vi "Measurement Logic.vi"(8 "error in":errorcluster, 9 "measurement configuration":T2, 10 "measure call context in":refnum<class "Measure Call Context.lvclass">, 11 "Stop OOB Server UE":refnum<user-event>) -> (0 "error out":errorcluster, 1 "measurement results":T1 {"Scanned Addresses" format="%.0x"}, 2 "measure call context out":refnum<class "Measure Call Context.lvclass">)   [LabVIEW 2025, in "I2C Bus Monitor.lvclass"]
doc: "Contains the core logic for executing the measurement."
uses:
  I2C Bus Monitor.lvclass
  <vilib>/Plug-In SDKs/Measurements/Measure Call Context/Measure Call Context.lvclass
  Measurement Configuration.ctl
  Measurement Results.ctl
  Typedefs/Logic Data.ctl
  Typedefs/State.ctl
  <instrlib>/FlexRIO/CSI-2/v2/FPGA/Types/Timestamp ID.ctl
  SubVIs/I2C Message Buffer - Create.vi
  SubVIs/I2C Message Buffer - Enqueue.vi
  SubVIs/I2C Message Buffer - Check.vi
  SubVIs/Error Global.vi
  SubVIs/I2C Message Buffer - Destroy.vi
  OOB Data Transfer/OOB Data Transfer.lvlib
  <instrlib>/_niInstr/Basic Elements/v1/FPGA/niInstr Basic Elements v1 FPGA.lvlib
  <instrlib>/FlexRIO/CSI-2/v2/FPGA/NI CSI-2 API FPGA v2.lvlib
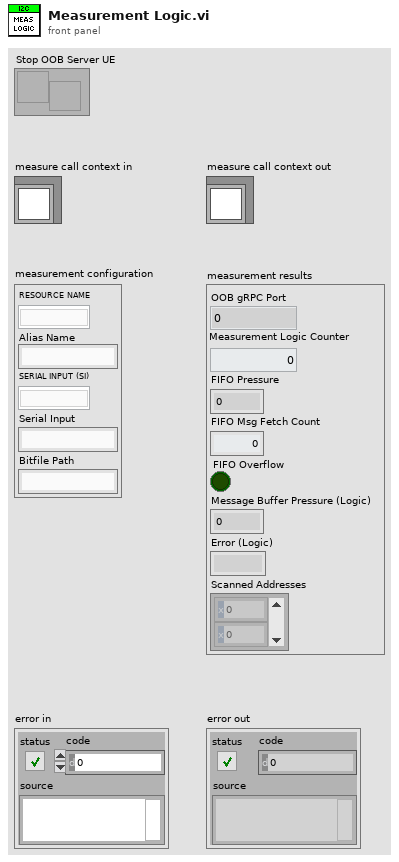
[diagram p1: front panel]
types:
  T1 = typedef "I2C Bus Monitor.lvclass/Measurement Results.ctl" = cluster{"OOB gRPC Port":i32, "Measurement Logic Counter":i32, "FIFO Pressure":u32, "FIFO Msg Fetch Count":i32, "FIFO Overflow":bool, "Message Buffer Pressure (Logic)":i32, "Error (Logic)":string, "Scanned Addresses":i32[]}
  T2 = typedef "I2C Bus Monitor.lvclass/Measurement Configuration.ctl" = cluster{"RESOURCE NAME":u32, "Alias Name":string, "SERIAL INPUT (SI)":u32, "Serial Input":string, "Bitfile Path":string}
  T3 = typedef "I2C Bus Monitor.lvclass/Logic Data.ctl" = cluster{"State":T4, "FPGA Ref":refnum<k20>, "Timestamp ID":T5, "Results":T1}
  T4 = typedef "I2C Bus Monitor.lvclass/State.ctl" = enum16{"Init", "Exec", "Results", "Error", "Close"}
  T5 = typedef "NI CSI-2 API FPGA v2.lvlib/Timestamp ID.ctl" = enum8{"SI0 LLP", "SI1 LLP", "SI2 LLP", "SI3 LLP", "SI4 LLP", "SI5 LLP", "SI6 LLP", "SI7 LLP", "SO0 LLP", "SO1 LLP", "SO2 LLP", "SO3 LLP", "SO4 LLP", "SO5 LLP", "SO6 LLP", "SO7 LLP", "Ser0 GPIO Bank", "Ser1 GPIO Bank", "Ser2 GPIO Bank", "Ser3 GPIO Bank", "Ser4 GPIO Bank", "Ser5 GPIO Bank", "Ser6 GPIO Bank", "Ser7 GPIO Bank", "Des0 GPIO Bank", "Des1 GPIO Bank", "Des2 GPIO Bank", "Des3 GPIO Bank", "Des4 GPIO Bank", "Des5 GPIO Bank", "Des6 GPIO Bank", "Des7 GPIO Bank", "User0", "User1", "User2", "User3", "User4", "User5", "User6", "User7", "User8", "User9", "User10", "User11", "User12", "User13", "User14", "User15", "User16", "User17", "User18", "User19", "User20", "User21", "User22", "User23", "User24", "User25", "User26", "User27", "User28", "User29", "User30", "User31"}
  T6 = typedef "OOB Data Transfer.lvlib/OOB to Logic Data.ctl" = cluster{"PauseResume":bool, "Export":string, "Scan Bus":bool, "I2C Script":cluster{"Send":bool, "Path":string}, "I2C CMD":cluster{"Send":bool, "SLAVE ADDR.":u8, "REG. ADDR.":u16, "DATA":u8, "R/W":bool}}
  T7 = cluster{"Send":bool, "SLAVE ADDR.":u8, "REG. ADDR.":u16, "DATA":u8, "R/W":bool}
  T8 = cluster{"Serial Input":string, "SLAVE ADDR.":u8, "REG. ADDR.":u16, "DATA":u8, "R/W":bool}
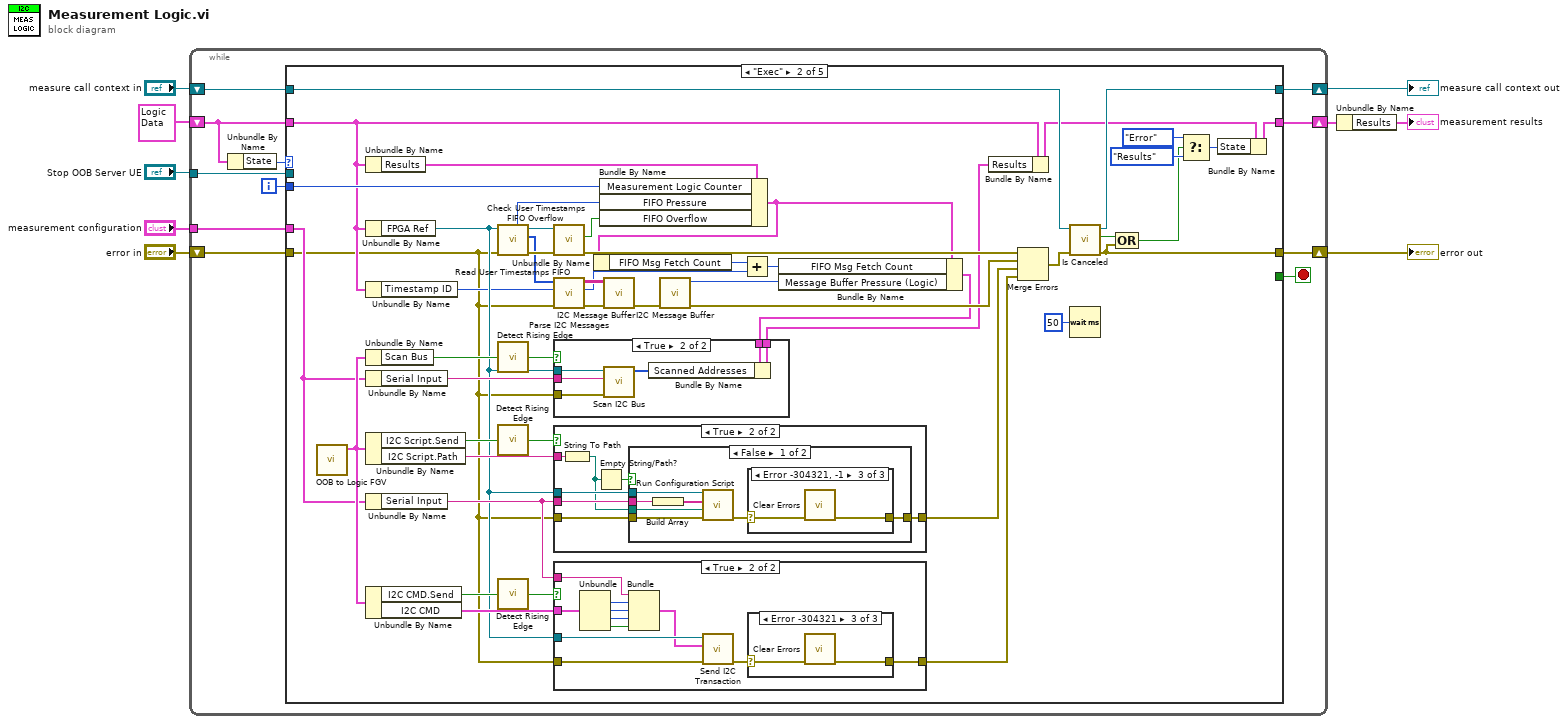
[diagram p0: block diagram]
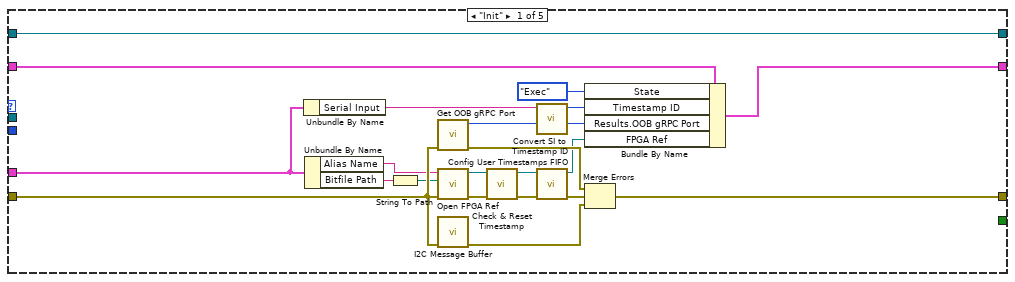
[diagram p2: hidden frame]
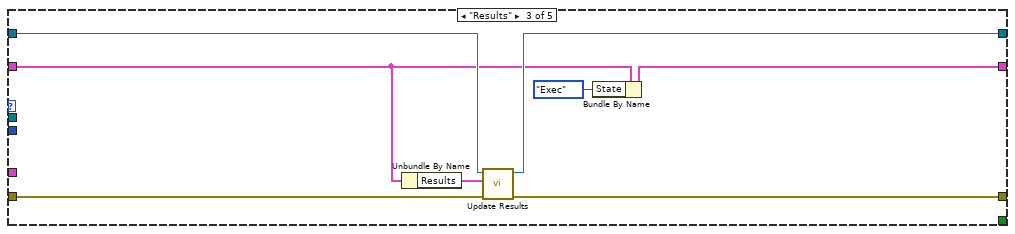
[diagram p11: hidden frame]
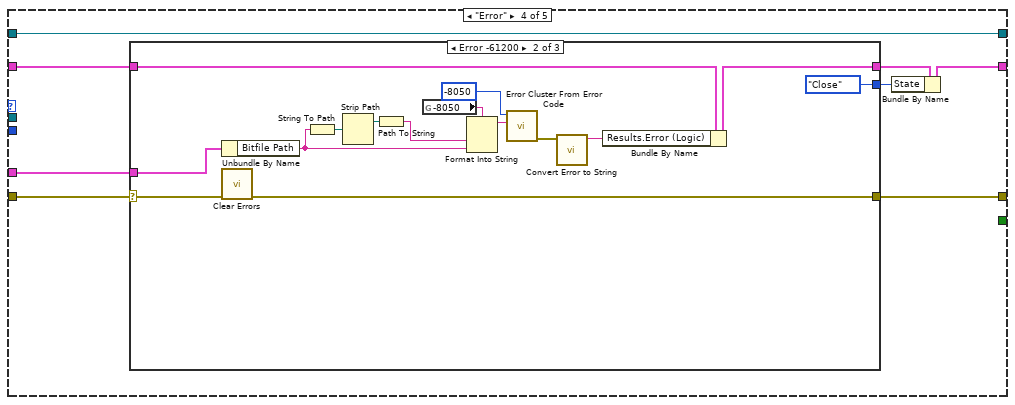
[diagram p12: hidden frame]
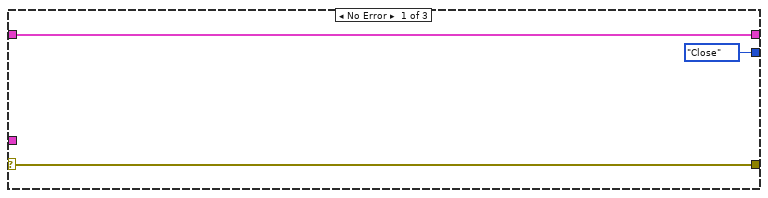
[diagram p13: hidden frame]
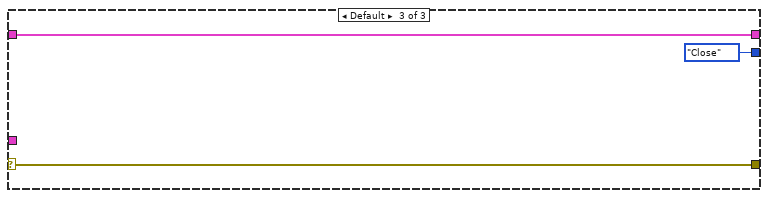
[diagram p14: hidden frame]
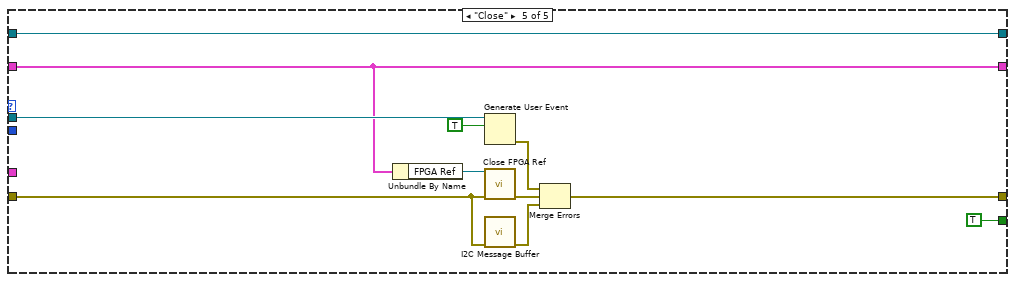
[diagram p15: hidden frame]
diagram:
  n1 = while {
    shift-right: [w15] -> w2
    shift-left: T3 {"State"=enum."Init", "FPGA Ref"=refnum, "Timestamp ID"=enum."SI0 LLP", "Results"={"OOB gRPC Port"=0, "Measurement Logic Counter"=0, "FIFO Pressure"=0, "FIFO Msg Fetch Count"=0, "FIFO Overflow"=FALSE, "Message Buffer Pressure (Logic)"=0, "Error (Logic)"="", "Scanned Addresses"=[]}} -> [w14]
    shift-right: [w10] -> w3
    shift-left: "error in" -> [w20]
    tunnel: "Stop OOB Server UE" -> [w18]
    tunnel: "measurement configuration" -> [w16]
    shift-right: [w11] -> w5
    shift-left: "measure call context in" -> [w17]
    i -> [w12]
    stop <- w19 stop-if-true
    n2 = Unbundle By Name(w14) -> ("State"=w13:T4)
    n3 = case shown="\"Exec\"" w13 {
      tunnel: w20 -> [w40 w44 w139 w148 w175]
      tunnel: [_ _ _ _ TRUE] -> w19
      tunnel: w18 -> [_ _ _ _ w179]
      tunnel: w17 -> [w22 w77 w137 w142 w180]
      tunnel: w16 -> [w25 w68 _ w143 _]
      tunnel: w14 -> [w39 w46 w135 w149 w171]
      tunnel: [w38 w79 w141 w145 w171] -> w15
      tunnel: w12 -> [_ w66 _ _ _]
      tunnel: [w26 w70 w138 w147 w174] -> w10
      tunnel: [w22 w76 w136 w142 w180] -> w11
      frame "Init" {
        n4 = Unbundle By Name(w25) -> ("Serial Input"=w36:string)
        n5 = Unbundle By Name(w25) -> ("Alias Name"=w31:string, "Bitfile Path"=w32:string)
        n6 = String To Path(string=w32) -> (path=w33:path)
        n7 = call "Get OOB gRPC Port.vi"("error in (no error)"=w40) -> ("error out"=w41:errorcluster, "OOB gRPC Port"=w21:i32)  [unwired: 9 in]
        n8 = call "Open FPGA Ref.vi"("error in (no error)"=w40, "Bitfile Path"=w33, "Device address"=w31) -> ("error out"=w34:errorcluster, "FPGA Ref out"=w29:refnum<k20>)  [unwired: 7 in]
        n9 = call-poly "I2C Message Buffer.vi"("error in (no error)"=w40) -> ("error out"=w27:errorcluster)  [unwired: 10 in]
        n10 = call "Check & Reset Timestamp.vi"("error in (no error)"=w34, "FPGA Ref in"=w29) -> ("error out"=w35:errorcluster, "FPGA Ref out"=w30:refnum<k20>)  [unwired: 8 in]
        n11 = call "Convert SI to Timestamp ID.vi"("SI Channel"=w36) -> ("Timestamp ID"=w23:T5)  [unwired: 10 in]
        n12 = call "Config User Timestamps FIFO.vi"("error in (no error)"=w35, "FPGA Ref in"=w30) -> ("error out"=w28:errorcluster, "FPGA Ref out"=w24:refnum<k20>)  [unwired: 8 in]
        n13 = Bundle By Name(cluster=w39, "State"=State."Exec", "Timestamp ID"=w23, "Results.OOB gRPC Port"=w21, "FPGA Ref"=w24) -> (w38:T3)
        n14 = Merge Errors(w41, w28, w27) -> (w26:errorcluster)
      }
      frame "Exec" {
        n15 = call "OOB to Logic FGV.vi"() -> ("OOB to Logic Data out"=w83:T6)  [unwired: 10 in, 1 out]
        n16 = Unbundle By Name(w46) -> ("Results"=w47:T1)
        n17 = Unbundle By Name(w46) -> ("FPGA Ref"=w60:refnum<k20>)
        n18 = Unbundle By Name(w46) -> ("Timestamp ID"=w53:T5)
        n19 = Unbundle By Name(w83) -> ("Scan Bus"=w61:bool)
        n20 = Unbundle By Name(w68) -> ("Serial Input"=w62:string)
        n21 = Unbundle By Name(w83) -> ("I2C Script.Send"=w88:bool, "I2C Script.Path"=w87:string)
        n22 = Unbundle By Name(w68) -> ("Serial Input"=w75:string)
        n23 = Unbundle By Name(w83) -> ("I2C CMD.Send"=w85:bool, "I2C CMD"=w82:T7)
        n24 = call "Read User Timestamps FIFO.vi"("error in (no error)"=w44, "FPGA Ref in"=w60) -> ("error out"=w90:errorcluster, "Data"=w54:u64[], "FPGA Ref out"=w81:refnum<k20>, "Elements Remaining"=w65:u32)  [unwired: 6 in]
        n25 = call <instrlib>:"Detect Rising Edge.vi"("signal"=w61) -> ("edge detected"=w51:bool)  [unwired: 14 in]
        n26 = call <instrlib>:"Detect Rising Edge.vi"("signal"=w88) -> ("edge detected"=w86:bool)  [unwired: 14 in]
        n27 = call <instrlib>:"Detect Rising Edge.vi"("signal"=w85) -> ("edge detected"=w84:bool)  [unwired: 14 in]
        n28 = call "Check User Timestamps FIFO Overflow.vi"("error in (no error)"=w90, "FPGA Ref in"=w81) -> ("error out"=w80:errorcluster, "User Timestamp FIFO Overflow"=w64:bool)  [unwired: 7 in, 1 out]
        n29 = call "Parse I2C Messages.vi"("error in (no error)"=w44, "Timestamp ID"=w53, "User Timestamps"=w54) -> ("error out"=w56:errorcluster, "Count"=w50:i32, "I2C Messages"=w55:string[][])  [unwired: 6 in]
        n30 = case shown="True" w86 {
          tunnel: w87 -> [_ w120]
          tunnel: w44 -> [w114 w119]
          tunnel: w60 -> [_ w121]
          tunnel: w75 -> [_ w118]
          tunnel: [w114 w117] -> w63
          frame False {
          }
          frame True {
            n31 = String To Path(string=w120) -> (path=w115:path)
            n32 = Empty String/Path?(string/path=w115) -> (empty?=w116:bool)
            n33 = case shown="False" w116 {
              tunnel: w121 -> [w126 _]
              tunnel: w115 -> [w124 _]
              tunnel: w119 -> [w128 w133]
              tunnel: w118 -> [w127 _]
              tunnel: [w122 w133] -> w117
              frame False {
                n34 = Build Array(w127) -> (w125:string[])
                n35 = call "Run Configuration Script.vi"("error in (no error)"=w128, "configuration script"=w124, "serial channels"=w125, "fpga interface in"=w126) -> ("error out"=w123:errorcluster)  [unwired: 6 in, 1 out]
                n36 = case shown="Error -304321, -1" w123 {
                  selector: w123 -> [w129 w130 w132]
                  tunnel: [w129 w130 w131] -> w122
                  frame No Error {
                  }
                  frame Default {
                  }
                  frame Error {
                    n37 = call <vilib>:"Clear Errors.vi"("error in (no error)"=w132) -> ("error out"=w131:errorcluster)  [unwired: 5 in, 1 out]
                  }
                }
              }
              frame True {
              }
            }
          }
        }
        n38 = case shown="True" w84 {
          tunnel: w82 -> [_ w107]
          tunnel: w44 -> [w98 w108]
          tunnel: w60 -> [_ w109]
          tunnel: [w98 w99] -> w69
          tunnel: w75 -> [_ w102]
          frame False {
          }
          frame True {
            n39 = Unbundle(w107) -> ("SLAVE ADDR."=w106:u8, "REG. ADDR."=w105:u16, "DATA"=w104:u8, "R/W"=w103:bool)  [unwired: 1 out]
            n40 = Bundle("Serial Input"=w102, "SLAVE ADDR."=w106, "REG. ADDR."=w105, "DATA"=w104, "R/W"=w103) -> (w101:T8)  [unwired: 1 in]
            n41 = call "Send I2C Transaction.vi"("Error In"=w108, "I2C Command"=w101, "FPGA Ref in"=w109) -> ("Error Out"=w100:errorcluster)  [unwired: 6 in, 2 out]
            n42 = case shown="Error -304321" w100 {
              selector: w100 -> [w110 w111 w113]
              tunnel: [w110 w111 w112] -> w99
              frame No Error {
              }
              frame Default {
              }
              frame Error {
                n43 = call <vilib>:"Clear Errors.vi"("error in (no error)"=w113) -> ("error out"=w112:errorcluster)  [unwired: 5 in, 1 out]
              }
            }
          }
        }
        n44 = Bundle By Name(cluster=w47, "Measurement Logic Counter"=w66, "FIFO Pressure"=w65, "FIFO Overflow"=w64) -> (w45:T1)
        n45 = Unbundle By Name(w45) -> ("FIFO Msg Fetch Count"=w48:i32)
        n46 = call-poly "I2C Message Buffer.vi"("error in (no error)"=w56, "I2C Messages"=w55) -> ("error out"=w57:errorcluster)  [unwired: 9 in]
        n47 = call-poly "I2C Message Buffer.vi"("error in (no error)"=w57) -> ("error out"=w52:errorcluster, "# elements in queue"=w58:i32)  [unwired: 9 in]
        n48 = Add(x=w48, y=w50) -> (x+y=w49:i32)
        n49 = Bundle By Name(cluster=w45, "FIFO Msg Fetch Count"=w49, "Message Buffer Pressure (Logic)"=w58) -> (w43:T1)
        n50 = case shown="True" w51 {
          tunnel: w62 -> [_ w97]
          tunnel: w60 -> [_ w96]
          tunnel: w44 -> [_ w94]
          tunnel: w43 -> [w91 w93]
          tunnel: [w91 w92] -> w42
          frame False {
          }
          frame True {
            n51 = call "Scan I2C Bus.vi"("error in (no error)"=w94, "Serial Input"=w97, "FPGA Ref"=w96) -> ("Scanned Addresses"=w95:i32[])  [unwired: 7 in, 1 out]
            n52 = Bundle By Name(cluster=w93, "Scanned Addresses"=w95) -> (w92:T1)
          }
        }
        n53 = Bundle By Name(cluster=w46, "Results"=w42) -> (w67:T3)
        n54 = Merge Errors(w80, w52, w63, w69) -> (w71:errorcluster)
        n55 = call <vilib>:"Is Canceled.vi"("error in"=w71, "measure call context in"=w77) -> ("error out"=w70:errorcluster, "is canceled?"=w89:bool, "measure call context out"=w76:refnum<class "Measure Call Context.lvclass">)  [unwired: 7 in]
        n56 = Wait (ms)(milliseconds to wait=u32 50) -> ()  [unwired: 1 out]
        n57 = Compound Arithmetic op=OR(w89, w70) -> (w72:bool)
        n58 = Select(t=State."Error" ("State"), s=w72, f=State."Results") -> (s? t:f=w74:T4)
        n59 = Bundle By Name(cluster=w67, "State"=w74) -> (w79:T3)
      }
      frame "Results" {
        n60 = Unbundle By Name(w135) -> ("Results"=w134:T1)
        n61 = call <vilib>:"Update Results.vi"("error in"=w139, "measurement results"=w134, "measure call context in"=w137) -> ("error out"=w138:errorcluster, "measure call context out"=w136:refnum<class "Measure Call Context.lvclass">)  [unwired: 7 in]
        n62 = Bundle By Name(cluster=w135, "State"=State."Exec") -> (w141:T3)
      }
      frame "Error" {
        n63 = case shown="Error -61200" w148 {
          selector: w148 -> [w151 w164 w170]
          tunnel: w149 -> [w152 w159 w168]
          tunnel: [w152 w166 w168] -> w144
          tunnel: [w151 w163 w170] -> w147
          tunnel: [State."Close" ("State") State."Close" ("State") State."Close" ("State")] -> w146
          tunnel: w143 -> [_ w158 _]
          frame No Error {
          }
          frame Error {
            n64 = Unbundle By Name(w158) -> ("Bitfile Path"=w154:string)
            n65 = call <vilib>:"Clear Errors.vi"("error in (no error)"=w164) -> ("error out"=w163:errorcluster)  [unwired: 5 in, 1 out]
            n66 = String To Path(string=w154) -> (path=w156:path)
            n67 = Strip Path(path=w156) -> (stripped path=w155:path)  [unwired: 1 out]
            n68 = Path To String(path=w155) -> (string=w153:string)
            n69 = global read "Error Global.vi" "-8050"() -> (w162:string)
            n70 = Format Into String(format string=w162, w153, w154) -> (resulting string=w161:string)  [unwired: 2 in, 1 out]
            n71 = call <vilib>:"Error Cluster From Error Code.vi"("error message (\"\")"=w161, "error code (0)"=-8050) -> ("error out"=w157:errorcluster)  [unwired: 7 in]
            n72 = call "Convert Error to String.vi"("error in (no error)"=w157) -> ("Error (Logic)"=w165:string)  [unwired: 10 in]
            n73 = Bundle By Name(cluster=w159, "Results.Error (Logic)"=w165) -> (w166:T3)
          }
          frame Default {
          }
        }
        n74 = Bundle By Name(cluster=w144, "State"=w146) -> (w145:T3)
      }
      frame "Close" {
        n75 = Unbundle By Name(w171) -> ("FPGA Ref"=w173:refnum<k20>)
        n76 = Generate User Event(user event=w179, event data cluster=TRUE ("event data")) -> (error out=w172:errorcluster)  [unwired: 2 in, 1 out]
        n77 = call "Close FPGA Ref.vi"("error in (no error)"=w175, "FPGA Ref in"=w173) -> ("error out"=w176:errorcluster)  [unwired: 9 in]
        n78 = call-poly "I2C Message Buffer.vi"("error in (no error)"=w175) -> ("error out"=w177:errorcluster)  [unwired: 10 in]
        n79 = Merge Errors(w172, w176, w177) -> (w174:errorcluster)
      }
    }
  }
  "error out" <- w3
  "measure call context out" <- w5
  n80 = Unbundle By Name(w2) -> ("Results"=→"measurement results":T1)
